vi "Agilent 3352X Series Arbitrary Waveform.vi"() -> ()   [LabVIEW 2010, in "AWG.lvlib"]
doc: "This example shows how to create then configure an arbitrary waveform."
uses:
  AWG.lvlib
  Instance           2 47Saved   Agilent 3352X Series Arbitrary Waveform .vi
  Instance           1 47Saved   Agilent 3352X Series Arbitrary Waveform .vi
  Agilent 3352X Series.lvlib
panel:
  in  "Offset (0.00 V)":dbl
  in  "Sample Rate (4000 Sa/s)":dbl=4000.0
  in  "Gain (0.1 Vpp)":dbl=0.1
  in  "Arbitrary Waveform Name":string="ARB1"
  in  "VISA resource name":refnum<visa-resource-name>
  # "(c) 2011-2015  National Instruments.  ALL RIGHTS RESERVED."
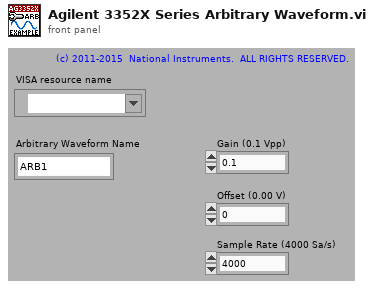
[diagram p1: front panel]
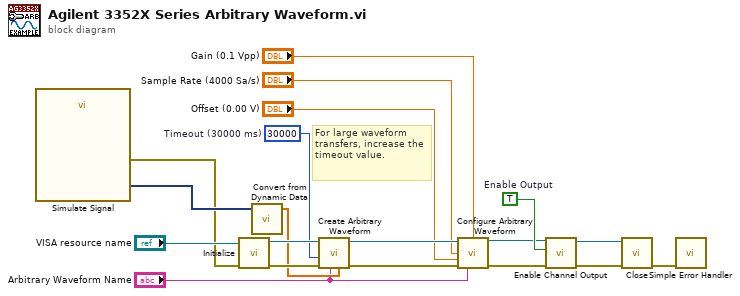
[diagram p0: block diagram]
diagram:
  w11 = TRUE  # Enable Output
  w1 = u32 30000  # Timeout (30000 ms)
  # "For large waveform transfers, increase the timeout value."
  n1 = call "Simulate Signal"() -> ("Sine with Uniform Noise"=w19:dynamicdata, "error out"=w17:errorcluster)  [unwired: 8 in, 6 out]
  n2 = call "Initialize.vi"("error in (no error)"=w17, "VISA resource name"="VISA resource name") -> ("error out"=w13:errorcluster, "VISA resource name out"=w12:refnum<visa-resource-name>)  [unwired: 2 in, 6 out]
  n3 = call "Convert from Dynamic Data"("Dynamic Data Type"=w19) -> ("Array"=w3:dbl[])  [unwired: 3 out]
  n4 = call "Create Arbitrary Waveform.vi"("Arbitrary Waveform Data"=w3, "Arbitrary Waveform Name (ARB1)"="Arbitrary Waveform Name", "error in (no error)"=w13, "Timeout (10000 ms)"=w1, "VISA resource name"=w12) -> ("error out"=w9:errorcluster, "VISA resource name out"=w10:refnum<visa-resource-name>)  [unwired: 2 in, 3 out]
  n5 = call "Configure Arbitrary Waveform.vi"("VISA resource name"=w10, "Amplitude (0.1 Vpp)"="Gain (0.1 Vpp)", "Sample Rate (40000 Sa/s)"="Sample Rate (4000 Sa/s)", "Offset (0 V)"="Offset (0.00 V)", "error in (no error)"=w9, "Arbitrary Waveform (ARB1)"="Arbitrary Waveform Name") -> ("VISA resource name out"=w7:refnum<visa-resource-name>, "error out"=w8:errorcluster)  [unwired: 4 in, 4 out]
  n6 = call "Enable Channel Output.vi"("error in (no error)"=w8, "Enable Output (T: Enable)"=w11, "VISA resource name"=w7) -> ("error out"=w15:errorcluster, "VISA resource name out"=w14:refnum<visa-resource-name>)  [unwired: 2 in, 5 out]
  n7 = call "Close.vi"("error in (no error)"=w15, "VISA resource name"=w14) -> ("error out"=w16:errorcluster)  [unwired: 9 out]
  n8 = call <vilib>:"Simple Error Handler.vi"("error in (no error)"=w16) -> ()  [unwired: 1 in, 8 out]
